vi "Format Fiducial Data.vi"(6 "Path Fiducials":T6(array[cluster]), 7 "Procedure Type":T7, 8 "error in":errorcluster, 9 "Module-Chuck Fiducials":T8(array[cluster]), 10 "Worktable":refnum<class "WorkTable Class.lvclass">, 11 "Console Log in":refnum<class "Console Log.lvclass">) -> (0 "error out":errorcluster, 2 "Formatted Fiducial Data":string, 3 "Console Log out":refnum<class "Console Log.lvclass">)   [LabVIEW 2011, in "Console Log.lvclass"]
uses:
  Console Log.lvclass
  Shared Components/Utils/Type Definitions/Fiducial Image.ctl
  Shared Components/Vec3d Class/Vec3d Class.lvclass
  Shared Components/Utils/Type Definitions/Physical Image.ctl
  <vilib>/vision/Image Controls.llb/IMAQ Image.ctl
  Shared Components/Utils/Type Definitions/Fiducial with Source.ctl
  Shared Components/WorkTable Class/WorkTable Class.lvclass
  Shared Components/WorkTable Class/Type Definitions/Worktable_Mode.ctl
  Shared Components/Utils/Type Definitions/Part Fiducials.ctl
  Shared Components/Config Manager Class/Type Definitions/Part Type.ctl
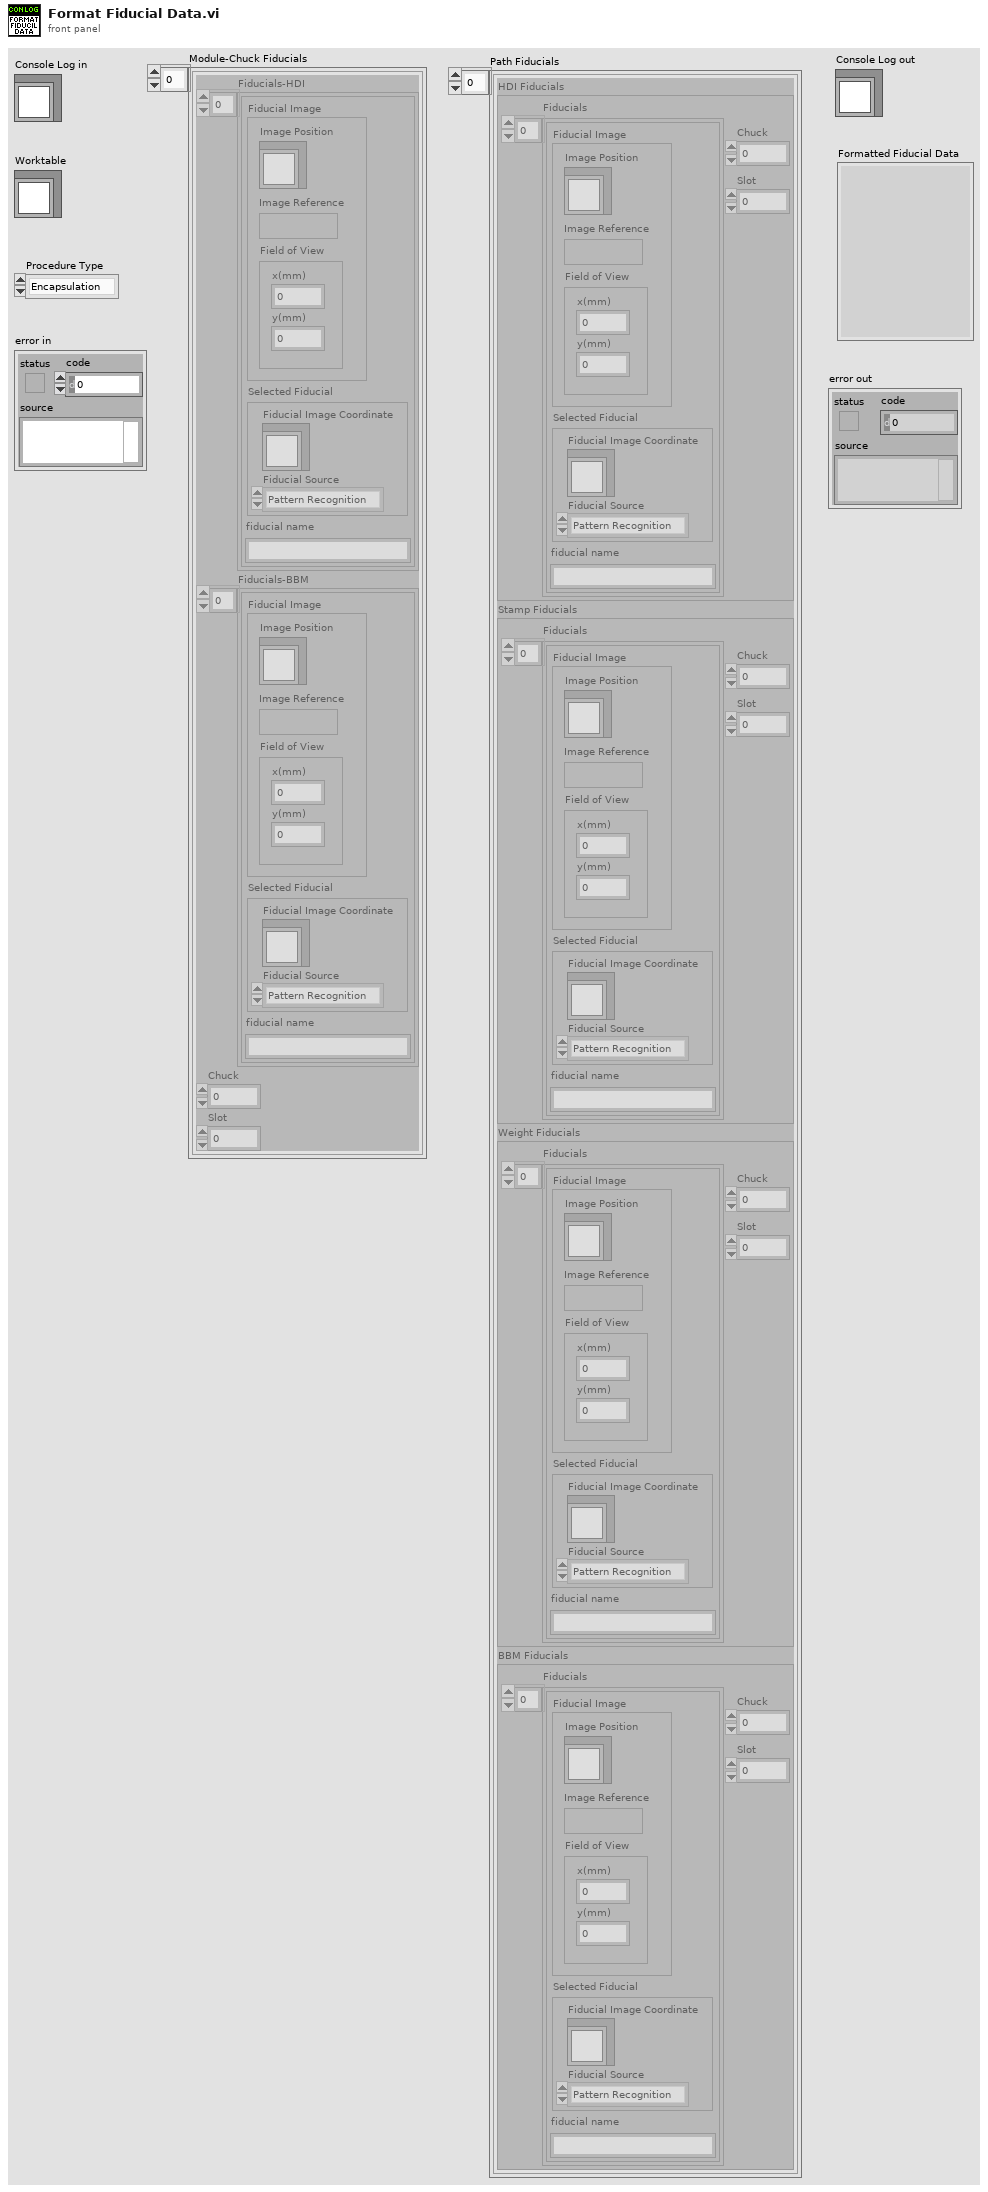
[diagram p1: front panel]
types:
  T1 = typedef "Part Fiducials.ctl" = cluster{"Fiducials":T2[], "Chuck":i32, "Slot":i32}
  T2 = typedef "Fiducial Image.ctl" = cluster{"Fiducial Image":T3, "Selected Fiducial":T5, "fiducial name":string}
  T3 = typedef "Physical Image.ctl" = cluster{"Image Position":refnum<class "Vec3d Class.lvclass">, "Image Reference":T4, "Field of View":cluster{"x(mm)":dbl, "y(mm)":dbl}}
  T4 = typedef "IMAQ Image.ctl" = refnum<image>
  T5 = typedef "Fiducial with Source.ctl" = cluster{"Fiducial Image Coordinate":refnum<class "Vec3d Class.lvclass">, "Fiducial Source":enum16{"Pattern Recognition", "User", "Error", "Default"}}
  T6 = cluster{"HDI Fiducials":T1, "Stamp Fiducials":T1, "Weight Fiducials":T1, "BBM Fiducials":T1}[]
  T7 = typedef "Worktable_Mode.ctl" = enum16{"Encapsulation", "Gluing"}
  T8 = cluster{"Fiducials-HDI":T2[], "Fiducials-BBM":T2[], "Chuck":i32, "Slot":i32}[]
  T9 = typedef "Part Type.ctl" = enum16{"BBM", "HDI", "BARE HDI", "GLUERESERVOIR", "STAMP_1", "STAMP_2", "STAMP_3", "STAMP_4", "STAMP_5", "WEIGHT_1", "WEIGHT_2", "WEIGHT_3", "WEIGHT_4", "WEIGHT_5", "WEIGHT_6", "WEIGHT_7", "WEIGHT_8", "PICKER_TOOL", "GRABER_TOOL"}
  T10 = typedef "Worktable_Module Slot.ctl" = cluster{"Slot State":enum16{"Empty", "Bare HDI", "Unglued", "Stamped", "PartOnTop", "Weighted", "Unpotted", "Potted"}, "BBM Type":enum16{"None", "BBM", "GlassSlide"}, "HDI Type":enum16{"None", "HDI", "Polyimide"}, "Vacuum Channel":u8, "Location/Orientation BBM":T11, "Location/Orientation HDI":T11, "S/N":string}
  T11 = typedef "Position_Orientation.ctl" = cluster{"Center":refnum<class "Vec3d Class.lvclass">, "Orientation":refnum<class "Orient3d Class.lvclass">}
  T12 = typedef "Worktable_Stamp.ctl" = cluster{"Stamp State":enum16{"Empty", "Populated", "Used"}, "Location/Orientation":T11, "Stamp Type":T13}
  T13 = typedef "Stamp Type.ctl" = enum16{"Stamp 1", "Stamp 2", "Stamp 3", "Stamp 4", "Stamp 5"}
  T14 = typedef "Worktable_Weight.ctl" = cluster{"Weight State":enum16{"Empty", "Populated"}, "Weight Type":T15, "Location/Orientation":T11}
  T15 = typedef "Weight Type.ctl" = enum16{"Weight 1", "Weight 2", "Weight 3", "Weight 4", "Weight 5", "Weight 6", "Weight 7", "Weight 8"}
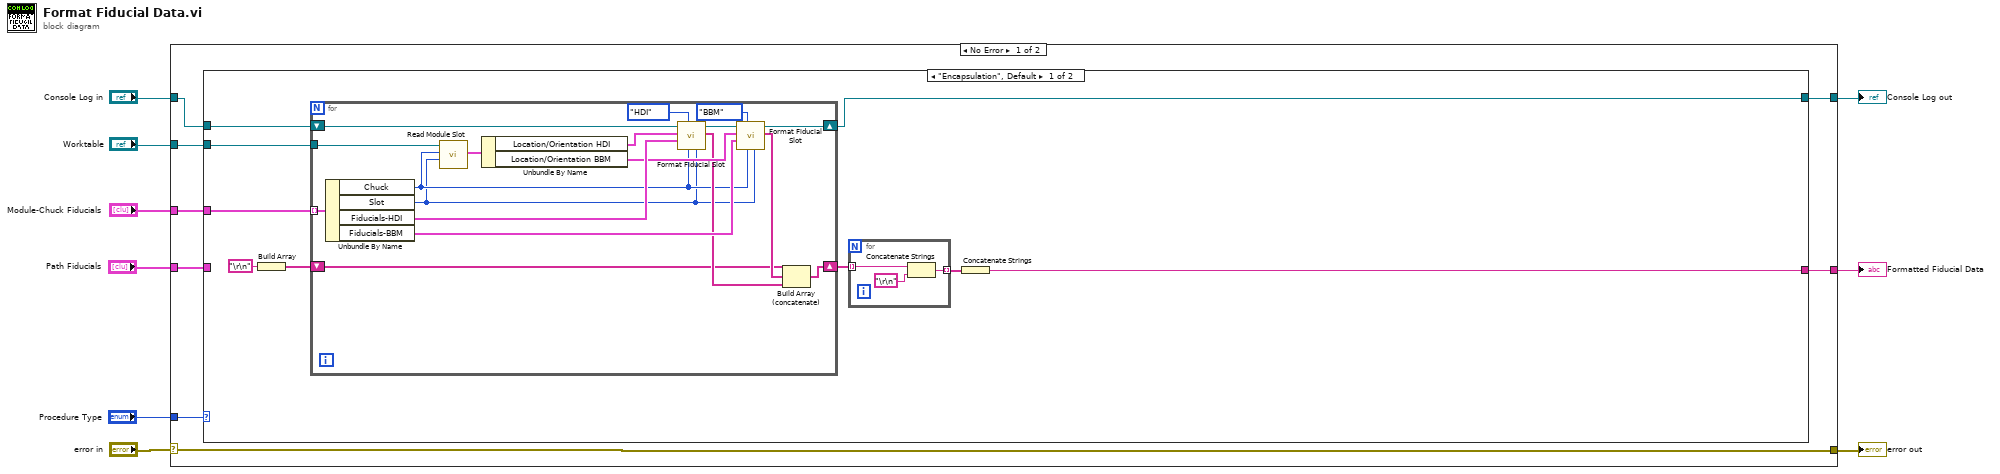
[diagram p0: block diagram]
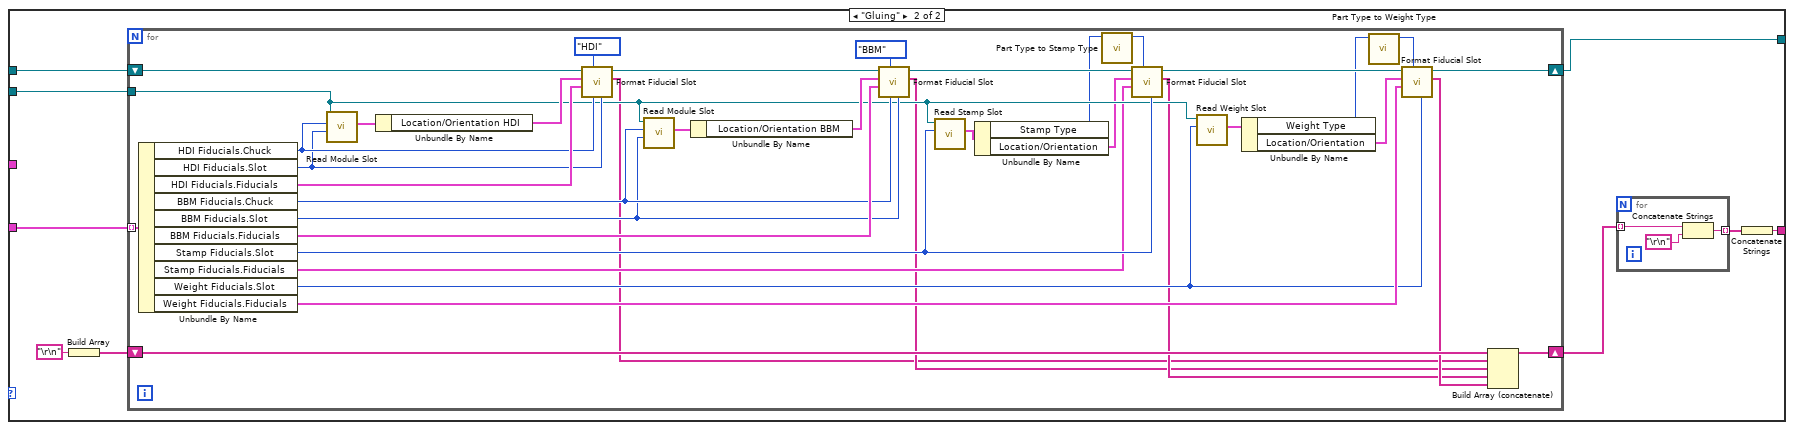
[diagram p2: hidden frame]
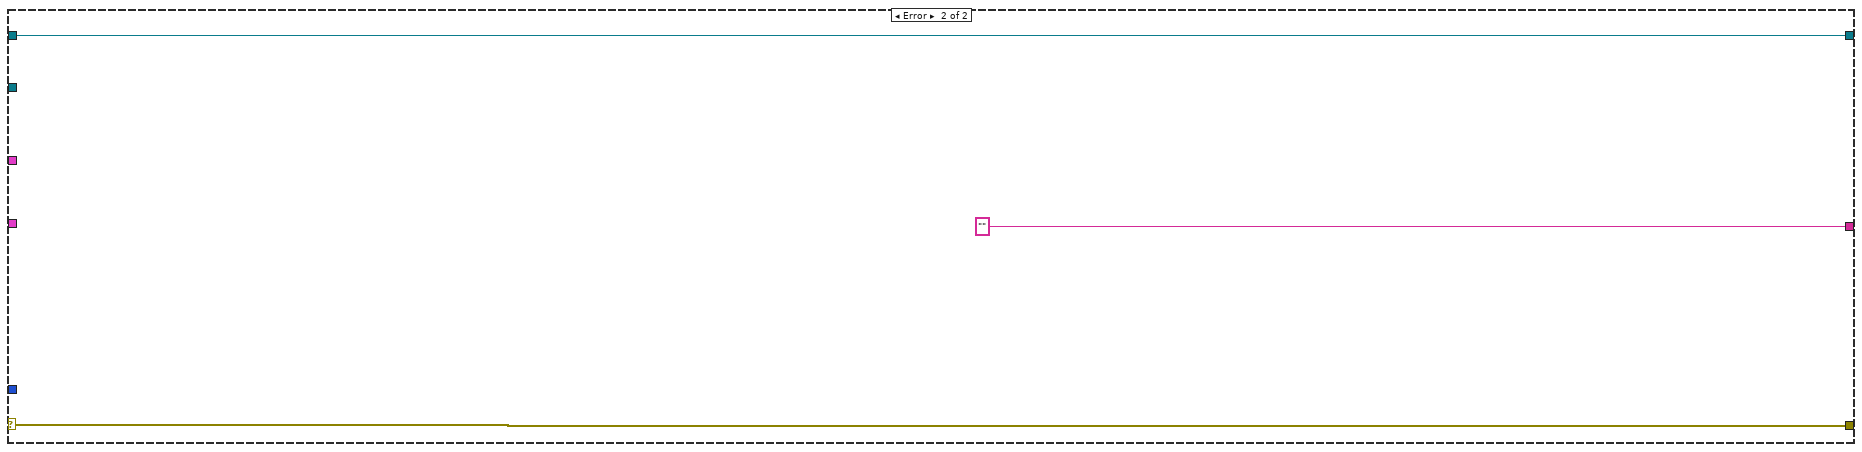
[diagram p3: hidden frame]
diagram:
  n1 = case shown="No Error" "error in" {
    selector: "error in" -> [w17 w99]
    tunnel: [w17 w99] -> w8
    tunnel: [w14 w98] -> w6
    tunnel: "Console Log in" -> [w15 w98]
    tunnel: "Module-Chuck Fiducials" -> [w10 _]
    tunnel: "Worktable" -> [w16 _]
    tunnel: [w13 ""] -> w3
    tunnel: "Procedure Type" -> [w12 _]
    tunnel: "Path Fiducials" -> [w11 _]
    frame No Error {
      n2 = case shown="\"Encapsulation\", Default" w12 {
        tunnel: w16 -> [w26 w56]
        tunnel: w15 -> [w25 w55]
        tunnel: [w24 w54] -> w14
        tunnel: [w21 w51] -> w13
        tunnel: w11 -> [_ w48]
        tunnel: w10 -> [w18 _]
        frame "Encapsulation", Default {
          n3 = Build Array("\r\n") -> (w19:string[])
          n4 = for {
            tunnel: w18 -> [w46] mode=indexing
            tunnel: w26 -> [w47]
            shift-right: [w40] -> w24
            shift-left: w25 -> [w42]
            shift-right: [w34] -> w23
            shift-left: w19 -> [w35]
            n5 = Unbundle By Name(w46) -> ("Chuck"=w33:i32, "Slot"=w32:i32, "Fiducials-HDI"=w43:T2[], "Fiducials-BBM"=w38:T2[])
            n6 = call-dynamic "Read Module Slot.vi"("slot"=w32, "chuck"=w33, "WorkTable in"=w47) -> ("Module Slot"=w45:T10)  [unwired: 6 in, 2 out]
            n7 = Unbundle By Name(w45) -> ("Location/Orientation HDI"=w44:T11, "Location/Orientation BBM"=w39:T11)
            n8 = call "Format Fiducial Slot.vi"("Slot"=w32, "Chuck"=w33, "Part Type"=Part_Type."HDI", "Fiducials"=w43, "Location/Orientation"=w44, "Console Log in"=w42) -> ("Array"=w36:string[], "Console Log out"=w41:refnum<class "Console Log.lvclass">)  [unwired: 3 in, 1 out]
            n9 = call "Format Fiducial Slot.vi"("Slot"=w32, "Chuck"=w33, "Part Type"=Part_Type."BBM", "Fiducials"=w38, "Location/Orientation"=w39, "Console Log in"=w41) -> ("Array"=w37:string[], "Console Log out"=w40:refnum<class "Console Log.lvclass">)  [unwired: 3 in, 1 out]
            n10 = Build Array (concatenate)(w35, w37, w36) -> (w34:string[])
          }
          n11 = for {
            tunnel: w23 -> [w29] mode=indexing
            tunnel: [w28] -> w22 mode=indexing
            n12 = Concatenate Strings(w29, "\r\n") -> (w28:string)
          }
          n13 = Concatenate Strings(w22) -> (w21:string)
        }
        frame "Gluing" {
          n14 = Build Array("\r\n") -> (w49:string[])
          n15 = for {
            tunnel: w56 -> [w75]
            shift-right: [w69] -> w54
            shift-left: w55 -> [w93]
            shift-right: [w90] -> w53
            shift-left: w49 -> [w91]
            tunnel: w48 -> [w85] mode=indexing
            n16 = Unbundle By Name(w85) -> ("HDI Fiducials.Chuck"=w89:i32, "HDI Fiducials.Slot"=w88:i32, "HDI Fiducials.Fiducials"=w94:T2[], "BBM Fiducials.Chuck"=w79:i32, "BBM Fiducials.Slot"=w78:i32, "BBM Fiducials.Fiducials"=w84:T2[], "Stamp Fiducials.Slot"=w76:i32, "Stamp Fiducials.Fiducials"=w73:T2[], "Weight Fiducials.Slot"=w70:i32, "Weight Fiducials.Fiducials"=w71:T2[])
            n17 = call-dynamic "Read Module Slot.vi"("slot"=w88, "chuck"=w89, "WorkTable in"=w75) -> ("Module Slot"=w96:T10)  [unwired: 6 in, 2 out]
            n18 = Unbundle By Name(w96) -> ("Location/Orientation HDI"=w95:T11)
            n19 = call "Format Fiducial Slot.vi"("Slot"=w88, "Chuck"=w89, "Part Type"=Part_Type."HDI", "Fiducials"=w94, "Location/Orientation"=w95, "Console Log in"=w93) -> ("Array"=w60:string[], "Console Log out"=w92:refnum<class "Console Log.lvclass">)  [unwired: 3 in, 1 out]
            n20 = call-dynamic "Read Module Slot.vi"("slot"=w78, "chuck"=w79, "WorkTable in"=w75) -> ("Module Slot"=w83:T10)  [unwired: 6 in, 2 out]
            n21 = Unbundle By Name(w83) -> ("Location/Orientation BBM"=w82:T11)
            n22 = call "Format Fiducial Slot.vi"("Slot"=w78, "Chuck"=w79, "Part Type"=Part_Type."BBM", "Fiducials"=w84, "Location/Orientation"=w82, "Console Log in"=w92) -> ("Array"=w61:string[], "Console Log out"=w80:refnum<class "Console Log.lvclass">)  [unwired: 3 in, 1 out]
            n23 = call "Read Stamp Slot.vi"("Stamp Slot"=w76, "WorkTable Class in"=w75) -> ("Stamp Slot"=w77:T12)  [unwired: 7 in, 2 out]
            n24 = Unbundle By Name(w77) -> ("Stamp Type"=w66:T13, "Location/Orientation"=w67:T11)
            n25 = call "Part Type to Stamp Type.vi"("Stamp Type"=w66) -> ("Part Type"=w81:T9)  [unwired: 9 in, 1 out]
            n26 = call "Format Fiducial Slot.vi"("Slot"=w76, "Part Type"=w81, "Fiducials"=w73, "Location/Orientation"=w67, "Console Log in"=w80) -> ("Array"=w62:string[], "Console Log out"=w74:refnum<class "Console Log.lvclass">)  [unwired: 4 in, 1 out]
            n27 = call "Read Weight Slot.vi"("weight slot"=w70, "WorkTable Class in"=w75) -> ("Weight Slot"=w72:T14)  [unwired: 7 in, 2 out]
            n28 = Unbundle By Name(w72) -> ("Weight Type"=w64:T15, "Location/Orientation"=w65:T11)
            n29 = call "Part Type to Weight Type.vi"("Weight Type"=w64) -> ("Part Type"=w68:T9)  [unwired: 9 in, 1 out]
            n30 = call "Format Fiducial Slot.vi"("Slot"=w70, "Part Type"=w68, "Fiducials"=w71, "Location/Orientation"=w65, "Console Log in"=w74) -> ("Array"=w63:string[], "Console Log out"=w69:refnum<class "Console Log.lvclass">)  [unwired: 4 in, 1 out]
            n31 = Build Array (concatenate)(w91, w60, w61, w62, w63) -> (w90:string[])
          }
          n32 = for {
            tunnel: w53 -> [w59] mode=indexing
            tunnel: [w58] -> w52 mode=indexing
            n33 = Concatenate Strings(w59, "\r\n") -> (w58:string)
          }
          n34 = Concatenate Strings(w52) -> (w51:string)
        }
      }
    }
    frame Error {
    }
  }
  "error out" <- w8
  "Console Log out" <- w6
  "Formatted Fiducial Data" <- w3
